vi "PID version.vi"() -> ()   [LabVIEW 2009, in "Varian Magnet.lvclass"]
uses:
  Varian Magnet.lvclass
  <vilib>/DAQmx/create/channels.llb/DAQmx Create Channel (AO-Voltage-Basic).vi
  <vilib>/DAQmx/create/channels.llb/DAQmx Create Channel (AI-Voltage-Basic).vi
  <vilib>/DAQmx/write.llb/DAQmx Write (Analog DBL 1Chan 1Samp).vi
  <vilib>/Analysis/NI_AALBase.lvlib
panel:
  in  "On":bool
  out "Actual Amps":dbl
  out "Waveform Chart 3":dynamicdata(graph)
  out "Waveform Chart 2":dynamicdata(graph)
  in  "KD":dbl
  in  "KI":dbl
  in  "KP":dbl
  out "Tesla":dbl(knob) scale=0.0..1.25
  in  "Field Desired (T)":dbl min=0.0 max=1.25 step=0.001
  out "Amps Desired":dbl
  out "Waveform Chart":dbl(graph)
  out "Amps":dbl(knob) scale=0.0..1.5
  out "Raw voltage":dbl format="%0.4f"
  in  "stop":bool
  in  "data":dbl min=-9.0 max=9.0 format="%0.2f"
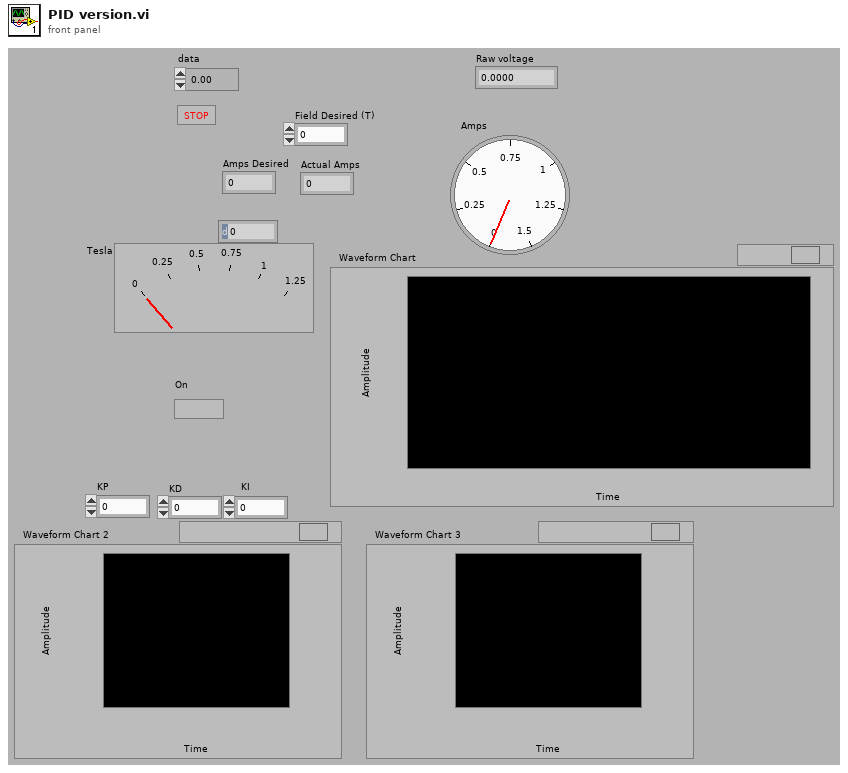
[diagram p1: front panel]
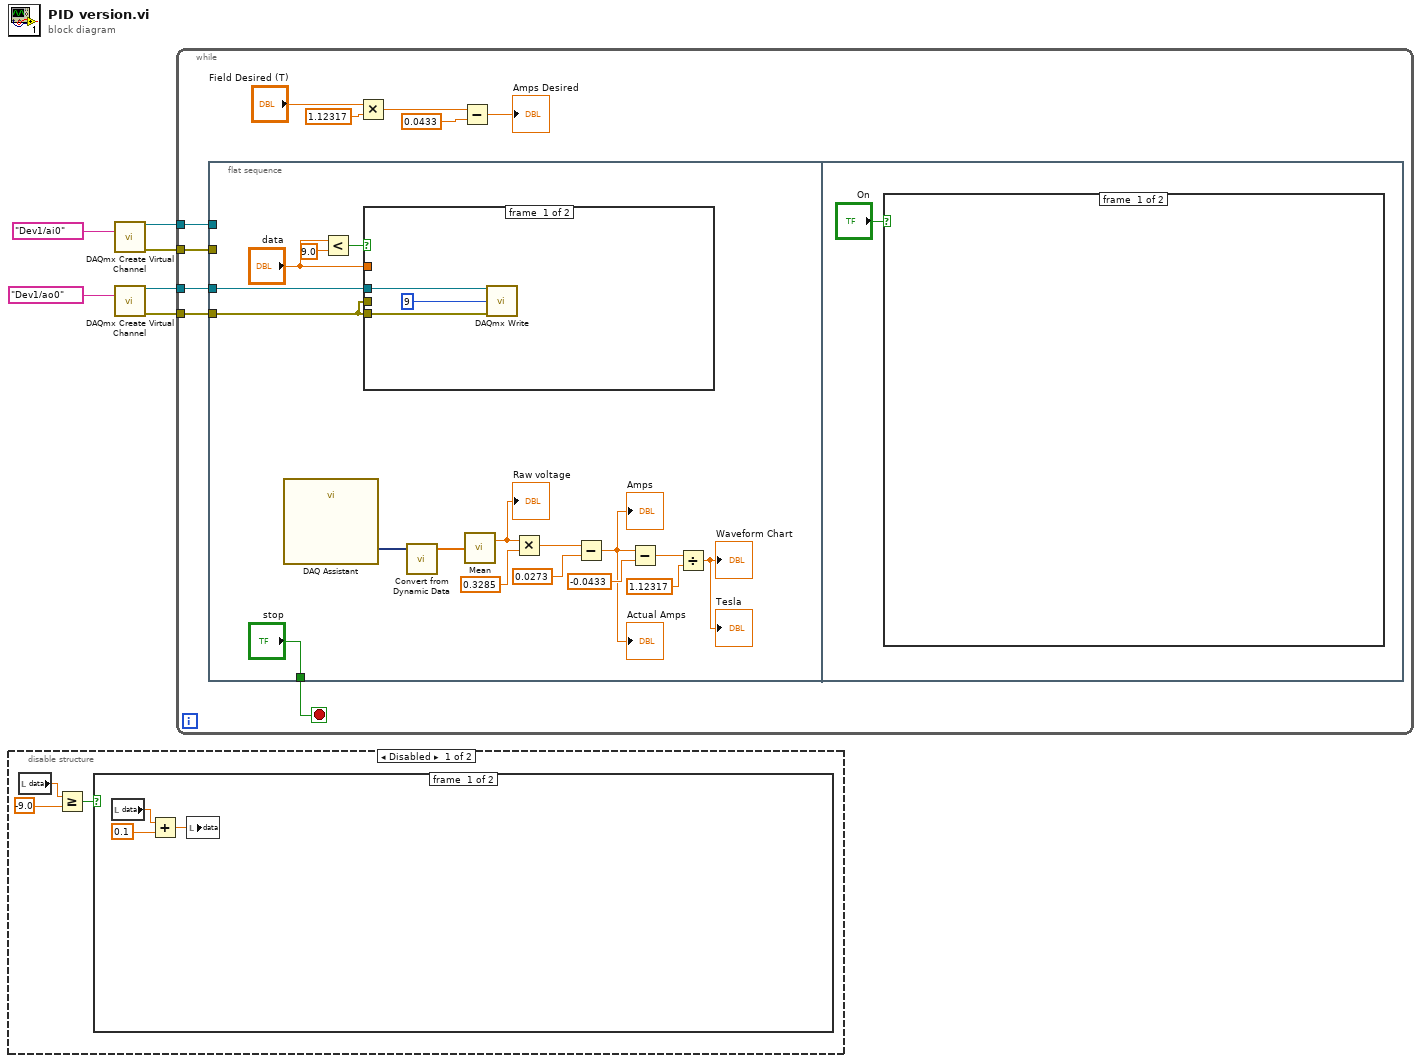
[diagram p0: block diagram]
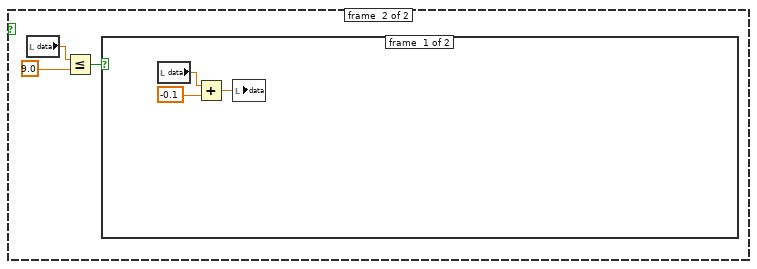
[diagram p2: hidden frame]
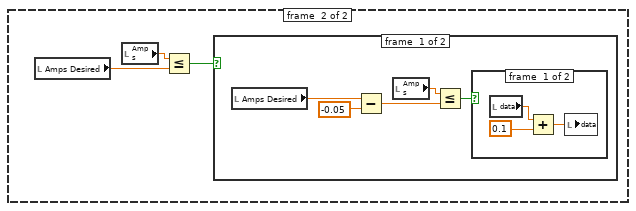
[diagram p3: hidden frame]
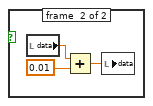
[diagram p4: hidden frame]
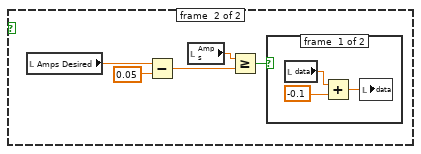
[diagram p5: hidden frame]
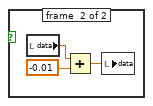
[diagram p6: hidden frame]
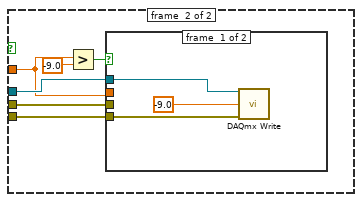
[diagram p8: hidden frame]
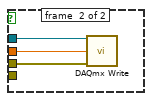
[diagram p9: hidden frame]
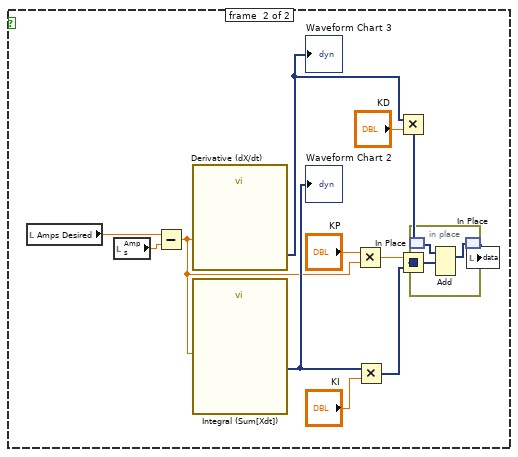
[diagram p10: hidden frame]
diagram:
  n1 = disable-structure shown="Disabled" {
    frame #0 {
      n2 = local read "data"() -> (w8:dbl)
      n3 = Greater Or Equal?(x=w8, y=-9.0) -> (x >= y?=w7:bool)
      n4 = case shown="True" w7 {
        frame #0 {
          n5 = local read "data"() -> (w11:dbl)
          n6 = Add(x=w11, y=0.1) -> (x+y=w10:dbl)
          n7 = local write "data"(w10) -> ()
        }
        frame #1 {
          n8 = local read "data"() -> (w15:dbl)
          n9 = Less Or Equal?(x=w15, y=9.0) -> (x <= y?=w13:bool)
          n10 = case shown="False" w13 {
            frame #0 {
              n11 = local read "data"() -> (w17:dbl)
              n12 = Add(x=w17, y=-0.1) -> (x+y=w16:dbl)
              n13 = local write "data"(w16) -> ()
            }
            frame #1 {
              n14 = local read "Amps Desired"() -> (w19:dbl)
              n15 = local read "Amps"() -> (w20:dbl)
              n16 = Less Or Equal?(x=w20, y=w19) -> (x <= y?=w21:bool)
              n17 = case shown="False" w21 {
                frame #0 {
                  n18 = local read "Amps Desired"() -> (w23:dbl)
                  n19 = Subtract(x=w23, y=-0.05) -> (x-y=w24:dbl)
                  n20 = local read "Amps"() -> (w26:dbl)
                  n21 = Less Or Equal?(x=w26, y=w24) -> (x <= y?=w25:bool)
                  n22 = case shown="False" w25 {
                    frame #0 {
                      n23 = local read "data"() -> (w28:dbl)
                      n24 = Add(x=w28, y=0.1) -> (x+y=w27:dbl)
                      n25 = local write "data"(w27) -> ()
                    }
                    frame #1 {
                      n26 = local read "data"() -> (w31:dbl)
                      n27 = Add(x=w31, y=0.01) -> (x+y=w30:dbl)
                      n28 = local write "data"(w30) -> ()
                    }
                  }
                }
                frame #1 {
                  n29 = local read "Amps Desired"() -> (w34:dbl)
                  n30 = Subtract(x=w34, y=0.05) -> (x-y=w35:dbl)
                  n31 = local read "Amps"() -> (w37:dbl)
                  n32 = Greater Or Equal?(x=w37, y=w35) -> (x >= y?=w36:bool)
                  n33 = case shown="True" w36 {
                    frame #0 {
                      n34 = local read "data"() -> (w39:dbl)
                      n35 = Add(x=w39, y=-0.1) -> (x+y=w38:dbl)
                      n36 = local write "data"(w38) -> ()
                    }
                    frame #1 {
                      n37 = local read "data"() -> (w42:dbl)
                      n38 = Add(x=w42, y=-0.01) -> (x+y=w41:dbl)
                      n39 = local write "data"(w41) -> ()
                    }
                  }
                }
              }
            }
          }
        }
      }
    }
    frame #1 {
    }
  }
  n40 = call-poly <vilib>:"DAQmx Create Virtual Channel.vi"("physical channels"=tag "Dev1/ai0") -> ("task out"=w3:refnum<k21>, "error out"=w2:errorcluster)  [unwired: 13 in]
  n41 = call-poly <vilib>:"DAQmx Create Virtual Channel.vi"("physical channels"=tag "Dev1/ao0") -> ("task out"=w5:refnum<k21>, "error out"=w4:errorcluster)  [unwired: 13 in]
  n42 = while {
    tunnel: w5 -> [w53]
    tunnel: w4 -> [w52]
    tunnel: w3 -> [w50]
    tunnel: w2 -> [w49]
    stop <- w51 stop-if-true
    n43 = flat-sequence {
      tunnel: w53 -> [w70]
      tunnel: w52 -> [w59]
      tunnel: ["stop"] -> w51
      tunnel: w50 -> [_]
      tunnel: w49 -> [_]
      frame #0 {
        n44 = call "DAQ Assistant"() -> ("data"=w68:dynamicdata)  [unwired: 17 in, 2 out]
        n45 = Less?(x="data", y=9.0) -> (x < y?=w56:bool)
        n46 = case shown="True" w56 {
          tunnel: w70 -> [w73 w79]
          tunnel: w59 -> [_ w78]
          tunnel: "data" -> [_ w74]
          tunnel: w59 -> [w72 w75]
          frame #0 {
            n47 = call-poly <vilib>:"DAQmx Write.vi"("task/channels in"=w73, "data"=9, "error in"=w72) -> ()  [unwired: 10 in, 3 out]
          }
          frame #1 {
            n48 = Greater?(x=w74, y=-9.0) -> (0:w77:bool)
            n49 = case shown="True" w77 {
              tunnel: w79 -> [w81 w85]
              tunnel: w78 -> [_ w84]
              tunnel: w74 -> [_ w83]
              tunnel: w75 -> [w82 _]
              frame #0 {
                n50 = call-poly <vilib>:"DAQmx Write.vi"("task/channels in"=w81, "data"=-9.0, "error in"=w82) -> ()  [unwired: 10 in, 3 out]
              }
              frame #1 {
                n51 = call-poly <vilib>:"DAQmx Write.vi"("task/channels in"=w85, "data"=w83, "error in"=w84) -> ()  [unwired: 10 in, 3 out]
              }
            }
          }
        }
        n52 = call "Convert from Dynamic Data"("Dynamic Data Type"=w68) -> ("Array"=w67:dbl[])  [unwired: 3 in]
        n53 = call <vilib>:"Mean.vi"("X"=w67) -> ("mean"=w66:dbl)  [unwired: 1 out]
        "Raw voltage" <- w66
        n54 = Multiply(x=w66, y=0.3285) -> (x*y=w64:dbl)
        n55 = Subtract(x=w64, y=0.0273) -> (x-y=w54:dbl)
        "Amps" <- w54
        "Actual Amps" <- w54
        n56 = Subtract(x=w54, y=-0.0433) -> (x-y=w60:dbl)
        n57 = Divide(x=w60, y=1.12317) -> (x/y=→"Waveform Chart" →"Tesla":dbl)
      }
      frame #1 {
        n58 = case shown="True" "On" {
          frame #0 {
          }
          frame #1 {
            n59 = local read "Amps Desired"() -> (w99:dbl)
            n60 = local read "Amps"() -> (w98:dbl)
            n61 = Subtract(x=w99, y=w98) -> (x-y=w87:dbl)
            n62 = call "Derivative (dX/dt)"("Signals"=w87) -> ("Result"=w88:dynamicdata)  [unwired: 1 in, 5 out]
            "Waveform Chart 3" <- w88
            n63 = call "Integral (Sum[Xdt])"("Signals"=w87) -> ("Result"=w89:dynamicdata)  [unwired: 1 in, 5 out]
            "Waveform Chart 2" <- w89
            n64 = Multiply(x="KP", y=w87) -> (x*y=w94:dbl)
            n65 = Multiply(x=w89, y="KI") -> (x*y=w93:dynamicdata)
            n66 = Multiply(x=w88, y="KD") -> (x*y=w91:dynamicdata)
            n67 = Add(x=w94, y=w93) -> (x+y=w92:dynamicdata)
            n68 = in-place {
              in-place-border: w92 -> [w102]
              n69 = in-place-match #1(w91) -> (w101:dynamicdata)
              n70 = Add(1:w102, 2:w101) -> (0:w100:dynamicdata)  [unwired: 1 in, 1 out]
              n71 = in-place-match #1(w100) -> (w90:dynamicdata)
            }
            n72 = local write "data"(w90) -> ()
          }
        }
      }
    }
    n73 = Multiply(x="Field Desired (T)", y=1.12317) -> (x*y=w48:dbl)
    n74 = Subtract(x=w48, y=0.0433) -> (x-y=→"Amps Desired":dbl)
  }
